vi "S-Curve Acceleration Centers.vi"(4 "v_f":dbl, 6 "v_i":dbl, 8 "t":dbl, 9 "j":dbl, 10 "a":dbl, 11 "v":dbl) -> (2 "c2":dbl, 3 "c1":dbl)   [LabVIEW 2025]
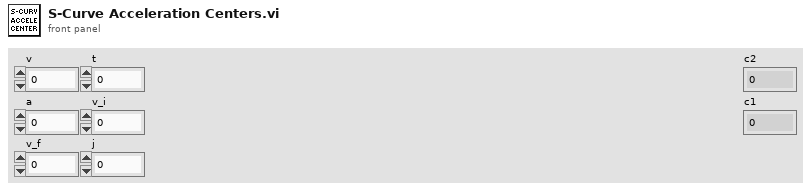
[diagram p1: front panel]
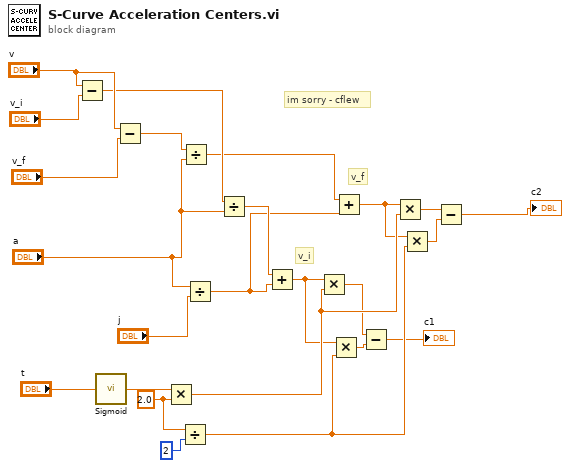
[diagram p0: block diagram]
diagram:
  w13 = 2.0 ("y")
  # "im sorry - cflew"
  # "v_i"
  # "v_f"
  n1 = Subtract(x="v", y="v_i") -> (x-y=w20:dbl)
  n2 = call "Sigmoid.vi"("x"="t") -> ("sigmoid(x)"=w14:dbl)
  n3 = Subtract(x="v", y="v_f") -> (x-y=w21:dbl)
  n4 = Multiply(x=w14, y=w13) -> (x*y=w11:dbl)
  n5 = Divide(x=w13, y=2) -> (x/y=w5:dbl)
  n6 = Divide(x=w21, y="a") -> (x/y=w16:dbl)
  n7 = Divide(x="a", y="j") -> (x/y=w15:dbl)
  n8 = Divide(x=w20, y="a") -> (x/y=w17:dbl)
  n9 = Add(x=w17, y=w15) -> (x+y=w6:dbl)
  n10 = Multiply(x=w6, y=w11) -> (x*y=w7:dbl)
  n11 = Multiply(x=w6, y=w5) -> (x*y=w4:dbl)
  n12 = Add(x=w16, y=w15) -> (x+y=w9:dbl)
  n13 = Subtract(x=w7, y=w4) -> (x-y=→"c1":dbl)
  n14 = Multiply(x=w9, y=w11) -> (x*y=w10:dbl)
  n15 = Multiply(x=w9, y=w5) -> (x*y=w8:dbl)
  n16 = Subtract(x=w10, y=w8) -> (x-y=→"c2":dbl)
